vi "K2450 Read Volt.vi"(8 "error in (no error)":errorcluster {"code" format="%.0x"}, 11 "VISA resource name":refnum<visa-resource-name>) -> (0 "error out":errorcluster {"code" format="%.0x"}, 2 "Voitage 2450":dbl, 3 "dup VISA Session":refnum<visa-resource-name>)   [LabVIEW 2019]
panel:
  # "Make sure unit is set up to read V\nsens:func \"volt\""
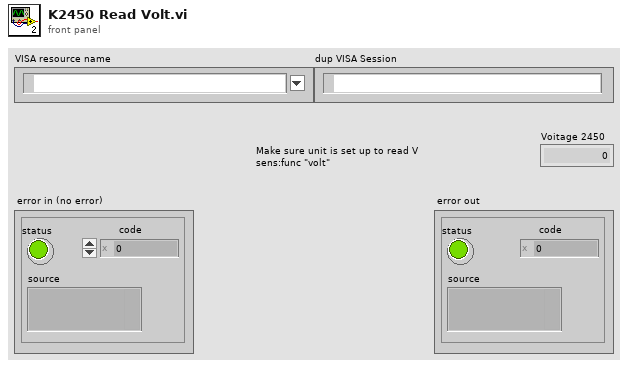
[diagram p1: front panel]
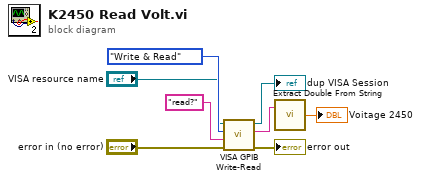
[diagram p0: block diagram]
diagram:
  n1 = call "VISA GPIB Write-Read.vi"("error in (no error)"="error in (no error)", "Command"="read?", "Action"=enum16{"Write", "Read", "Write & Read"}."Write & Read", "VISA resource name"="VISA resource name") -> ("error out"=→"error out":errorcluster, "String Returned"=w6:string, "dup VISA Session"=→"dup VISA Session":refnum<visa-resource-name>)  [unwired: 4 in, 1 out]
  n2 = call "Extract Double From String.vi"("string"=w6) -> ("floating pt. number"=→"Voitage 2450":dbl)  [unwired: 1 in, 2 out]
